vi "Shell and Tube Heat Exchanger.vi"() -> ()   [LabVIEW 2017]
uses:
  FlowSet S&THx.vi
  Level Set S&THx.vi
  Halt S&THx.vi
  Steam Set S&THx.vi
  <vilib>/addons/control/pid/pid.llb/PID Control Input Filter (DBL).vi
  <vilib>/addons/control/pid/pid.llb/PID Advanced (DBL).vi
  Flow Out S&THx.vi
  Level Out S&THx.vi
  Steam Out S&THx.vi
  <vilib>/addons/control/pid/NI_PID_pid.lvlib
panel:
  out "Last Time Write":dbl format="%#_13g"
  in  "Replace File":bool
  in  "Enable 5":bool
  in  "error in (no error)":errorcluster
  out "Makeup Flowrate":dbl caption="L/min"
  out "Makeup Temperature":dbl caption="C"
  in  "Td (Steam)":dbl caption="(min)"
  in  "Ti (Steam)":dbl=0.05 caption="(min)"
  in  "Kc (Steam)":dbl=0.5
  in  "Set Manual Valve Position (Steam Pressure)":dbl(slide) scale=0.0..100.0
  in  "Manual Control Override (Steam Pressure)":bool
  out "Steam Valve":dbl(slide) scale=0.0..100.0
  out "Steam Pressure":dbl=-37.335458390625 caption="psig" format="%.2f"
  in  "Steam Pressure Setpoint (psig)":dbl=10.0 min=0.0 max=45.0 format="%.2f"
  in  "Main Power":bool
  out "Tube-Side Pressure Drop":dbl=-3.685330554375 caption="psig"
  out "House Steam Pressure":dbl=-37.255405696875 caption="psig" format="%#.6g"
  in  "Td (Level)":dbl caption="(min)"
  in  "Ti (Level)":dbl=0.005 caption="(min)"
  in  "Kc (Level)":dbl=-75.0
  in  "Td (Flow)":dbl caption="(min)"
  in  "Ti (Flow)":dbl=0.036 caption="(min)"
  in  "Kc (Flow)":dbl=0.74
  in  "Set Manual Valve Position (Level)":dbl(slide) scale=0.0..100.0
  in  "Manual Control Override (Level)":bool=TRUE
  out "Level Control Valve":dbl(slide) scale=0.0..100.0
  out "Liquid Level in Tank":dbl=-0.5063459005125 format="%.2f"
  in  "Level Setpoint (ft)":dbl=1.5 min=0.0 max=2.0 format="%.2f"
  in  "Set Manual Valve Position (Flow)":dbl(slide)=100.0 scale=0.0..100.0
  in  "Manual Control Override (Flow)":bool=TRUE
  out "Flow Control Valve":dbl(slide)=100.0 scale=0.0..100.0
  out "Water Flowrate":dbl=-0.0021672099828720093 format="%.2f"
  in  "Flowrate Setpoint (GPM)":dbl=40.0 min=0.0 max=50.0 format="%.2f"
  in  "stop":bool
  out "Water Outlet Temperature":dbl=18.512494216488157 format="%.1f"
  out "Water Inlet Temperature":dbl=17.931811705329704 format="%.1f"
  in  "Pump Switch":bool
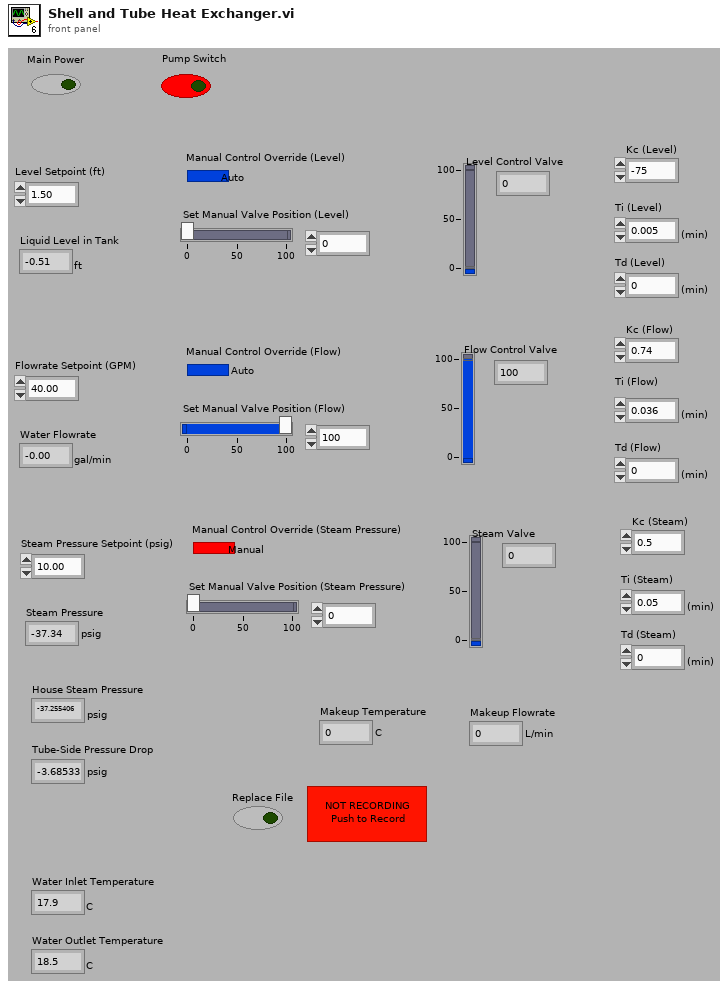
[diagram p1: front panel]
types:
  T1 = enum16{"open", "replace", "create", "open or create", "replace or create", "replace or create with confirmation"}
  T2 = cluster{"Kc (Flow)":dbl, "Ti (Flow)":dbl, "Td (Flow)":dbl}
  T3 = cluster{"Kc (Level)":dbl, "Ti (Level)":dbl, "Td (Level)":dbl}
  T4 = cluster{"Kc (Steam)":dbl, "Ti (Steam)":dbl, "Td (Steam)":dbl}
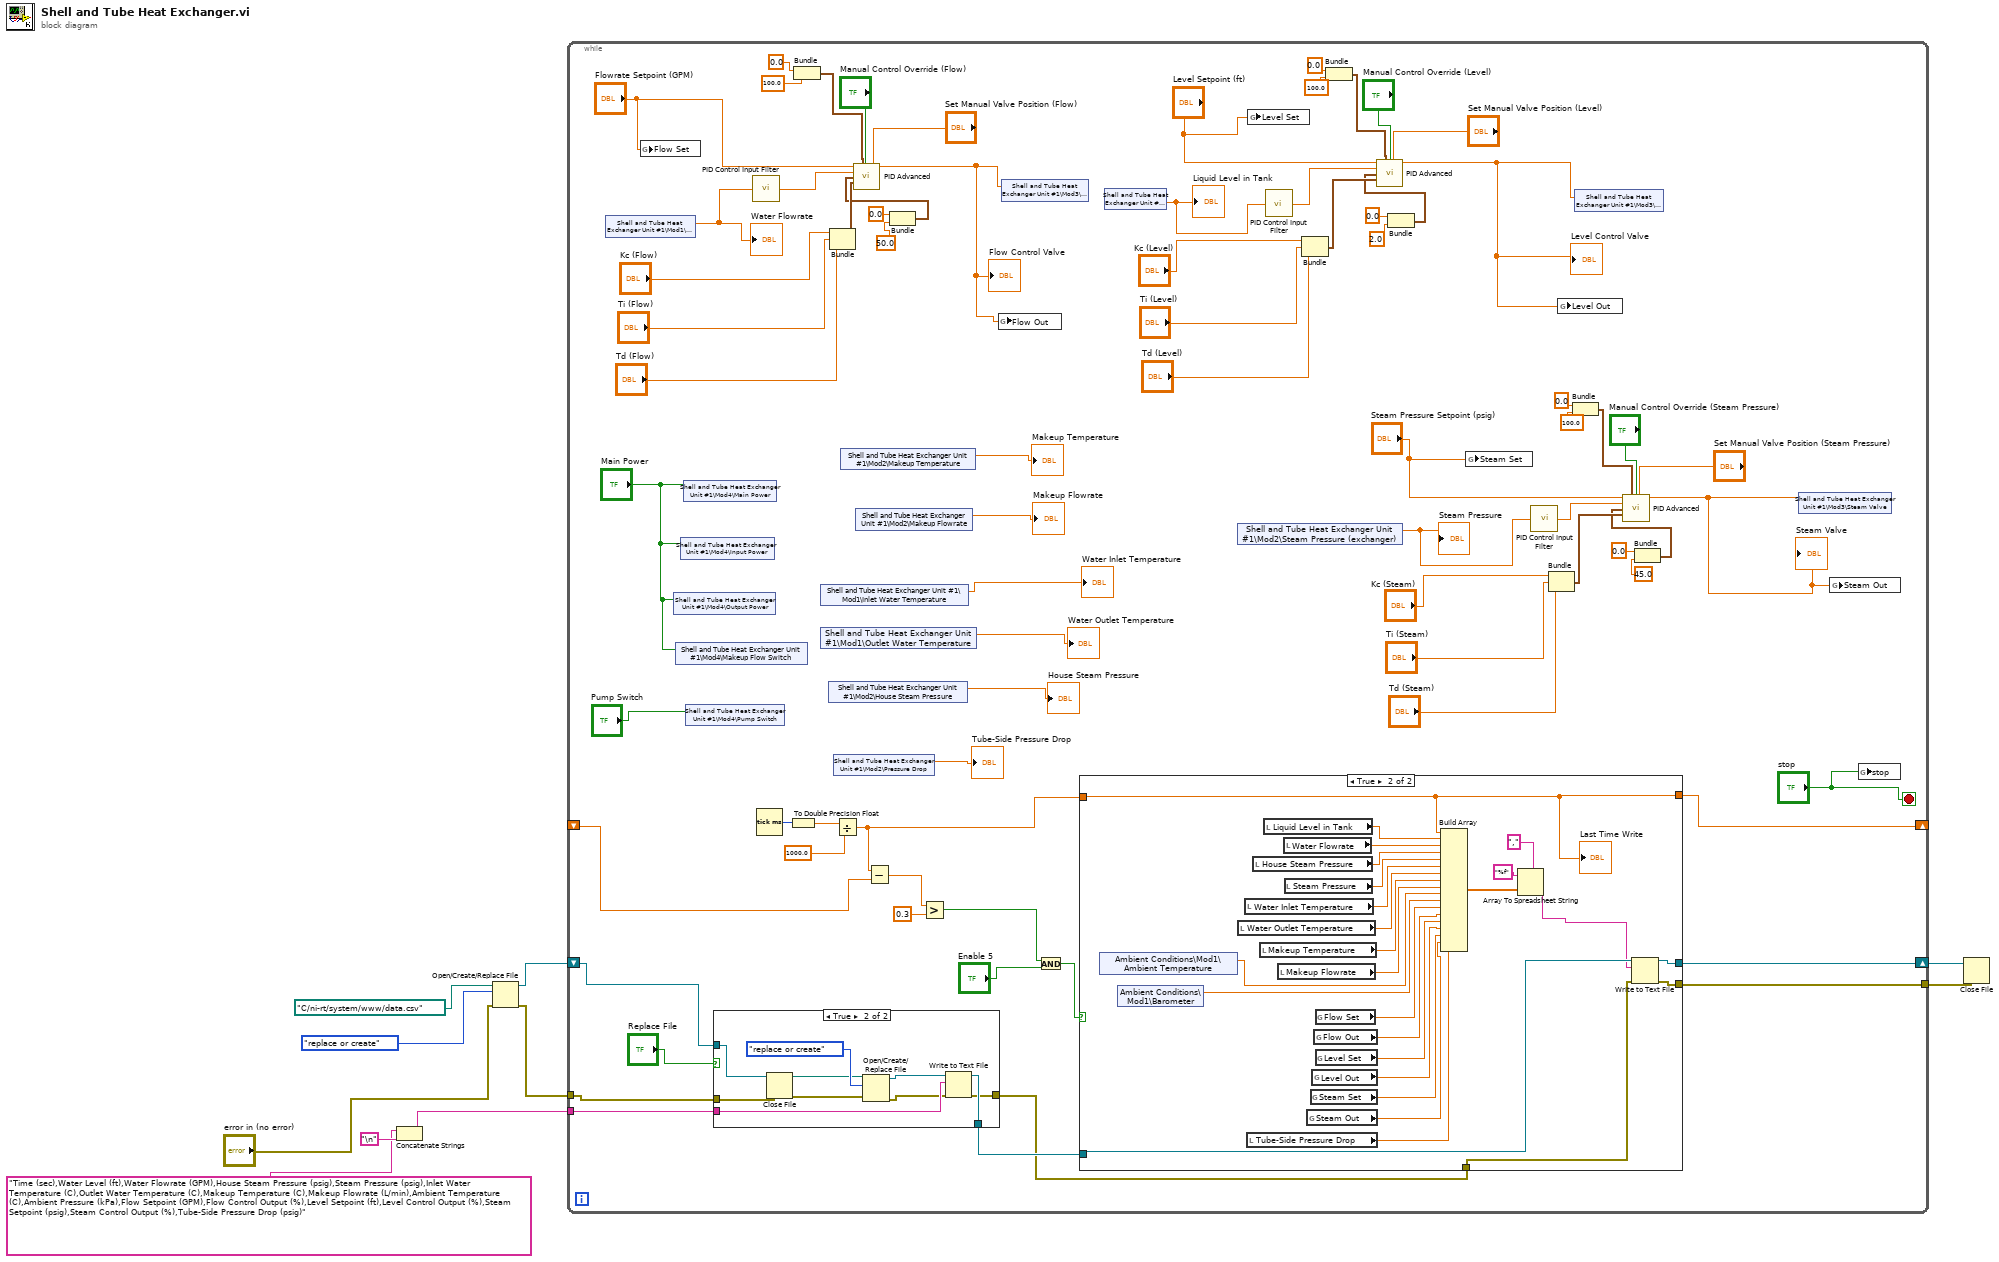
[diagram p0: block diagram]
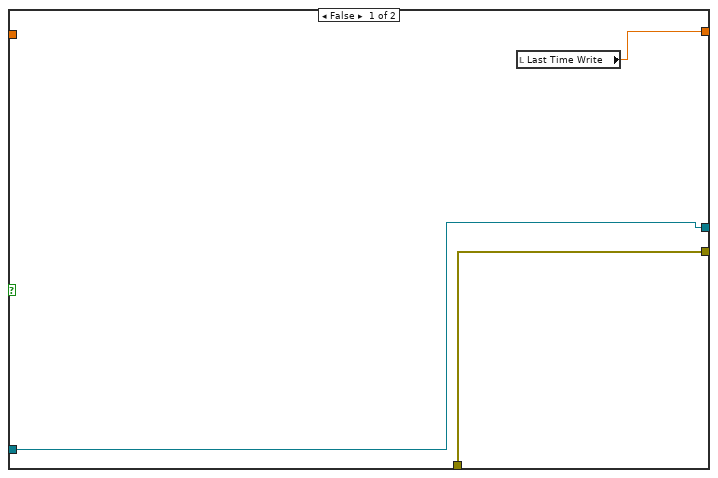
[diagram p3: hidden frame]
diagram:
  n1 = Concatenate Strings("Time (sec),Water Level (ft),Water Flowrate (GPM),House Steam Pressure (psig),Steam Pressure (psig),Inlet Water Temperature (C),Outlet Water Temperature (C),Makeup Temperature (C),Makeup Flowrate (L/min),Ambient Temperature (C),Ambient Pressure (kPa),Flow Setpoint (GPM),Flow Control Output (%),Level Setpoint (ft),Level Control Output (%),Steam Setpoint (psig),Steam Control Output (%),Tube-Side Pressure Drop (psig)", "\n") -> (w6:string)
  n2 = Open/Create/Replace File(file path (use dialog)=path "C:/ni-rt/system/www/data.csv" ("Filename"), error in="error in (no error)", operation (0:open)=T1."replace or create") -> (refnum out=w5:refnum<file>, error out=w2:errorcluster)  [unwired: 3 in, 1 out]
  n3 = while {
    tunnel: [w28] -> w9
    tunnel: w2 -> [w24]
    tunnel: w6 -> [w25]
    shift-right: [w29] -> w10
    shift-left: w5 -> [w22]
    shift-right: [w16] -> _
    shift-left: _ -> [w14]
    stop <- "stop" stop-if-true
    n4 = shared-variable "Shell and Tube Heat Exchanger Unit #1\\Mod1\\Water Flow"() -> (w35:dbl)  [unwired: 1 in, 1 out]
    "Water Flowrate" <- w35
    n5 = global write "FlowSet S&THx.vi" "Flow Set"("Flowrate Setpoint (GPM)") -> ()
    n6 = shared-variable "Shell and Tube Heat Exchanger Unit #1\\Mod4\\Output Power"("Main Power") -> ()  [unwired: 1 in, 1 out]
    n7 = shared-variable "Shell and Tube Heat Exchanger Unit #1\\Mod4\\Makeup Flow Switch"("Main Power") -> ()  [unwired: 1 in, 1 out]
    n8 = shared-variable "Shell and Tube Heat Exchanger Unit #1\\Mod4\\Input Power"("Main Power") -> ()  [unwired: 1 in, 1 out]
    n9 = shared-variable "Shell and Tube Heat Exchanger Unit #1\\Mod4\\Main Power"("Main Power") -> ()  [unwired: 1 in, 1 out]
    n10 = shared-variable "Shell and Tube Heat Exchanger Unit #1\\Mod4\\Pump Switch"("Pump Switch") -> ()  [unwired: 1 in, 1 out]
    n11 = case shown="True" "Replace File" {
      tunnel: [w87 w96] -> w26
      tunnel: w25 -> [_ w95]
      tunnel: w24 -> [w88 w92]
      tunnel: [w88 w93] -> w23
      tunnel: w22 -> [w87 w90]
      frame False {
      }
      frame True {
        n12 = Close File(refnum=w90, error in=w92) -> (path=w89:path, error out=w91:errorcluster)
        n13 = Open/Create/Replace File(file path (use dialog)=w89, error in=w91, operation (0:open)=T1."replace or create") -> (refnum out=w97:refnum<file>, error out=w94:errorcluster)  [unwired: 3 in, 1 out]
        n14 = Write to Text File(file (use dialog)=w97, text=w95, error in=w94) -> (refnum out=w96:refnum<file>, error out=w93:errorcluster)  [unwired: 1 in, 1 out]
      }
    }
    n15 = call-poly <vilib>:"PID Control Input Filter.vi"("input"=w35) -> ("output"=w34:dbl)  [unwired: 4 in]
    n16 = Tick Count (ms)() -> (millisecond timer value=w21:u32)
    n17 = To Double Precision Float(number=w21) -> (double precision float=w19:dbl)
    n18 = Bundle(0.0, 100.0) -> (w62:cluster{dbl, dbl})  [unwired: 1 in]
    n19 = shared-variable "Shell and Tube Heat Exchanger Unit #1\\Mod1\\Inlet Water Temperature"() -> (→"Water Inlet Temperature":dbl)  [unwired: 1 in, 1 out]
    n20 = shared-variable "Shell and Tube Heat Exchanger Unit #1\\Mod1\\Outlet Water Temperature"() -> (→"Water Outlet Temperature":dbl)  [unwired: 1 in, 1 out]
    n21 = shared-variable "Shell and Tube Heat Exchanger Unit #1\\Mod2\\House Steam Pressure"() -> (→"House Steam Pressure":dbl)  [unwired: 1 in, 1 out]
    n22 = Bundle("Kc (Flow)"="Kc (Flow)", "Ti (Flow)"="Ti (Flow)", "Td (Flow)"="Td (Flow)") -> (w82:T2)  [unwired: 1 in]
    n23 = shared-variable "Shell and Tube Heat Exchanger Unit #1\\Mod2\\Pressure Drop"() -> (→"Tube-Side Pressure Drop":dbl)  [unwired: 1 in, 1 out]
    n24 = Divide(x=w19, y=1000.0) -> (x/y=w15:dbl)
    n25 = shared-variable "Shell and Tube Heat Exchanger Unit #1\\Mod2\\Makeup Temperature"() -> (→"Makeup Temperature":dbl)  [unwired: 1 in, 1 out]
    n26 = shared-variable "Shell and Tube Heat Exchanger Unit #1\\Mod2\\Makeup Flowrate"() -> (→"Makeup Flowrate":dbl)  [unwired: 1 in, 1 out]
    n27 = Subtract(x=w15, y=w14) -> (x-y=w13:dbl)
    n28 = Bundle(0.0, 50.0) -> (w59:cluster{dbl, dbl})  [unwired: 1 in]
    n29 = call-poly <vilib>:"PID Advanced.vi"("setpoint"="Flowrate Setpoint (GPM)", "output range"=w62, "auto? (T)"="Manual Control Override (Flow)", "manual control"="Set Manual Valve Position (Flow)", "process variable"=w34, "setpoint range"=w59, "PID gains"=w82) -> ("output"=w69:dbl)  [unwired: 7 in, 1 out]
    "Flow Control Valve" <- w69
    n30 = Greater?(x=w13, y=0.3) -> (0:w12:bool)
    n31 = global write "Flow Out S&THx.vi" "Flow Out"(w69) -> ()
    n32 = shared-variable "Shell and Tube Heat Exchanger Unit #1\\Mod3\\Flow Valve"(w69) -> ()  [unwired: 1 in, 1 out]
    n33 = And(x=w12, y="Enable 5") -> (x .and. y?=w11:bool)
    n34 = case shown="True" w11 {
      tunnel: w26 -> [w100 w127]
      tunnel: [w100 w116] -> w29
      tunnel: [w101 w115] -> w28
      tunnel: w23 -> [w101 w114]
      tunnel: w15 -> [_ w102]
      tunnel: [w99 w102] -> w16
      frame False {
        n35 = local read "Last Time Write"() -> (w99:dbl)
      }
      frame True {
        n36 = shared-variable "Ambient Conditions\\Mod1\\Ambient Temperature"() -> (w104:dbl)  [unwired: 1 in, 1 out]
        n37 = shared-variable "Ambient Conditions\\Mod1\\Barometer"() -> (w103:dbl)  [unwired: 1 in, 1 out]
        n38 = local read "Water Outlet Temperature"() -> (w119:dbl)
        n39 = local read "Water Inlet Temperature"() -> (w120:dbl)
        n40 = local read "Tube-Side Pressure Drop"() -> (w107:dbl)
        n41 = local read "House Steam Pressure"() -> (w123:dbl)
        n42 = local read "Makeup Temperature"() -> (w118:dbl)
        n43 = local read "Liquid Level in Tank"() -> (w124:dbl)
        n44 = local read "Makeup Flowrate"() -> (w117:dbl)
        n45 = local read "Water Flowrate"() -> (w122:dbl)
        n46 = local read "Steam Pressure"() -> (w121:dbl)
        n47 = global read "Steam Out S&THx.vi" "Steam Out"() -> (w108:dbl)
        n48 = global read "Steam Set S&THx.vi" "Steam Set"() -> (w109:dbl)
        n49 = global read "Level Out S&THx.vi" "Level Out"() -> (w110:dbl)
        n50 = global read "Flow Out S&THx.vi" "Flow Out"() -> (w112:dbl)
        n51 = global read "FlowSet S&THx.vi" "Flow Set"() -> (w113:dbl)
        n52 = global read "Level Set S&THx.vi" "Level Set"() -> (w111:dbl)
        n53 = Build Array(w102, w124, w122, w123, w121, w120, w119, w118, w117, w104, w103, w113, w112, w111, w110, w109, w108, w107) -> (w125:dbl[])
        n54 = Array To Spreadsheet String(delimiter (Tab)=",", array=w125, 3:"%f" ("format string")) -> (spreadsheet string=w105:string)
        n55 = Write to Text File(file (use dialog)=w127, text=w105, error in=w114) -> (refnum out=w116:refnum<file>, error out=w115:errorcluster)  [unwired: 1 in, 1 out]
        "Last Time Write" <- w102
      }
    }
    n56 = shared-variable "Shell and Tube Heat Exchanger Unit #1\\Mod2\\Level"() -> (w30:dbl)  [unwired: 1 in, 1 out]
    "Liquid Level in Tank" <- w30
    n57 = shared-variable "Shell and Tube Heat Exchanger Unit #1\\Mod2\\Steam Pressure (exchanger)"() -> (w38:dbl)  [unwired: 1 in, 1 out]
    "Steam Pressure" <- w38
    n58 = global write "Level Set S&THx.vi" "Level Set"("Level Setpoint (ft)") -> ()
    n59 = call-poly <vilib>:"PID Control Input Filter.vi"("input"=w30) -> ("output"=w36:dbl)  [unwired: 4 in]
    n60 = Bundle("Kc (Level)"="Kc (Level)", "Ti (Level)"="Ti (Level)", "Td (Level)"="Td (Level)") -> (w84:T3)  [unwired: 1 in]
    n61 = Bundle(0.0, 100.0) -> (w65:cluster{dbl, dbl})  [unwired: 1 in]
    n62 = Bundle(0.0, 2.0) -> (w56:cluster{dbl, dbl})  [unwired: 1 in]
    n63 = call-poly <vilib>:"PID Advanced.vi"("setpoint"="Level Setpoint (ft)", "output range"=w65, "auto? (T)"="Manual Control Override (Level)", "manual control"="Set Manual Valve Position (Level)", "process variable"=w36, "setpoint range"=w56, "PID gains"=w84) -> ("output"=w41:dbl)  [unwired: 7 in, 1 out]
    "Level Control Valve" <- w41
    n64 = global write "Steam Set S&THx.vi" "Steam Set"("Steam Pressure Setpoint (psig)") -> ()
    n65 = call-poly <vilib>:"PID Control Input Filter.vi"("input"=w38) -> ("output"=w37:dbl)  [unwired: 4 in]
    n66 = Bundle("Kc (Steam)"="Kc (Steam)", "Ti (Steam)"="Ti (Steam)", "Td (Steam)"="Td (Steam)") -> (w51:T4)  [unwired: 1 in]
    n67 = global write "Level Out S&THx.vi" "Level Out"(w41) -> ()
    n68 = Bundle(0.0, 100.0) -> (w46:cluster{dbl, dbl})  [unwired: 1 in]
    n69 = shared-variable "Shell and Tube Heat Exchanger Unit #1\\Mod3\\Level Valve"(w41) -> ()  [unwired: 1 in, 1 out]
    n70 = Bundle(0.0, 45.0) -> (w43:cluster{dbl, dbl})  [unwired: 1 in]
    n71 = call-poly <vilib>:"PID Advanced.vi"("setpoint"="Steam Pressure Setpoint (psig)", "output range"=w46, "auto? (T)"="Manual Control Override (Steam Pressure)", "manual control"="Set Manual Valve Position (Steam Pressure)", "process variable"=w37, "setpoint range"=w43, "PID gains"=w51) -> ("output"=w40:dbl)  [unwired: 7 in, 1 out]
    "Steam Valve" <- w40
    n72 = shared-variable "Shell and Tube Heat Exchanger Unit #1\\Mod3\\Steam Valve"(w40) -> ()  [unwired: 1 in, 1 out]
    n73 = global write "Steam Out S&THx.vi" "Steam Out"(w40) -> ()
    n74 = global write "Halt S&THx.vi" "stop"("stop") -> ()
  }
  n75 = Close File(refnum=w10, error in=w9) -> ()  [unwired: 2 out]
